vi "register status change event.vi"(11 "generate status number":i32=100) -> (3 "status number":i32)   [LabVIEW 2017, in "testcase-documentation.lvclass"]
uses:
  testcase-documentation.lvclass
  src/user.lib/_NEVSTOP/Communicable State Machine(CSM)/_Support/Priority Queue/Priority Queue.lvclass/Priority Queue.ctl
  f9bca660-bddd-4266-99d8-d96952150cc2.vi
  src/user.lib/_NEVSTOP/Communicable State Machine(CSM)/_Support/Process/CSMP-Sync Call.vi
  src/user.lib/_NEVSTOP/Communicable State Machine(CSM)/Utility/uuid.vi
  src/user.lib/_NEVSTOP/Communicable State Machine(CSM)/Utility/Build Error Cluster.vi
  src/user.lib/_NEVSTOP/Communicable State Machine(CSM)/Utility/Trim Both Whitespace.vi
  src/user.lib/_NEVSTOP/Communicable State Machine(CSM)/AdvanceAPI/CSM - List Modules.vi
  src/user.lib/_NEVSTOP/Communicable State Machine(CSM)/_Support/CSMQ/_CSMObj-Message Check.vi
  src/user.lib/_NEVSTOP/Communicable State Machine(CSM)/_Support/CSMQ/_CSMObj-Enqueue Cross-Module Message.vi
  src/user.lib/_NEVSTOP/Communicable State Machine(CSM)/_Support/CSMQ/_CSMOFGV Get.vi
  src/user.lib/_NEVSTOP/Communicable State Machine(CSM)/_Support/Priority Queue/Enqueue Element.vi
  src/user.lib/_NEVSTOP/Communicable State Machine(CSM)/_Support/Error/CSM No Target Error.vi
  src/user.lib/_NEVSTOP/Communicable State Machine(CSM)/_Support/CSMQ/_CSMOFGV.vi
  src/user.lib/_NEVSTOP/Communicable State Machine(CSM)/_Support/Error/CSM Not Allowed Message.vi
  src/user.lib/_NEVSTOP/Communicable State Machine(CSM)/_Support/Error/CSM Target Error.vi
  src/user.lib/_NEVSTOP/Communicable State Machine(CSM)/_Support/Error/CSM Unhandled State Error.vi
  src/user.lib/_NEVSTOP/Communicable State Machine(CSM)/_Support/Error/CSM Target Timeout Error.vi
  src/user.lib/_NEVSTOP/Communicable State Machine(CSM)/_Support/FGV-BroadcastRegistry/global-CSMQ FGV Change Flag.vi
  src/user.lib/_NEVSTOP/Communicable State Machine(CSM)/Communicable State Machine.lvlib
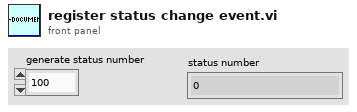
[diagram p1: front panel]
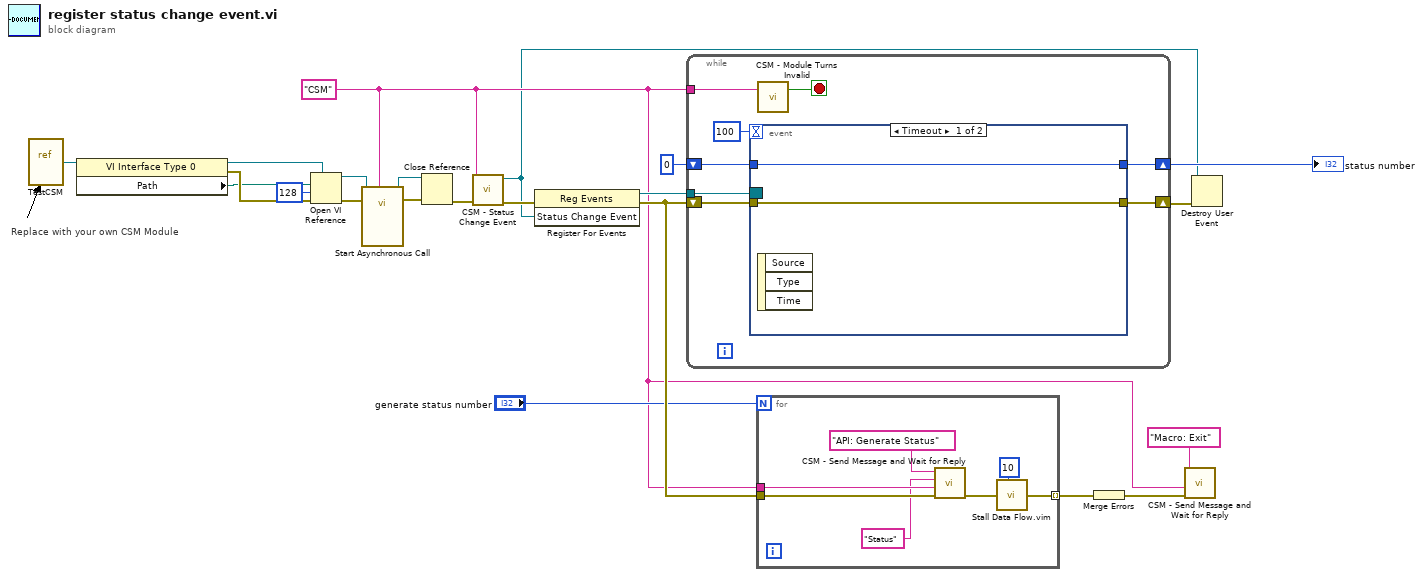
[diagram p0: block diagram]
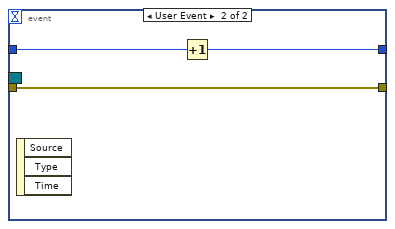
[diagram p2: hidden frame]
diagram:
  w6 = "CSM" ("Name(\"\" to use uuid)")
  # "Replace with your own CSM Module"
  n1 = vi-ref "TestCSM.vi"() -> (w15:refnum<vi>)
  n2 = property class="VI Interface Type 0"(reference=w15) -> (reference out=w19:refnum<vi>, error out=w17:errorcluster, "Path"=w16:path)  [unwired: 1 in]
  n3 = Open VI Reference(type specifier VI Refnum (for type only)=w19, vi path=w16, options=128, error in (no error)=w17) -> (vi reference=w18:refnum<vi>, error out=w14:errorcluster)  [unwired: 2 in]
  n4 = call-by-ref "Start Asynchronous Call"(reference=w18, error in=w14, "Name(\"\" to use uuid)"=w6) -> (reference out=w21:refnum<vi>, error out=w20:errorcluster)  [unwired: 11 in]
  n5 = Close Reference(reference=w21, error in (no error)=w20) -> (error out=w13:errorcluster)
  n6 = call "CSM - Status Change Event.vi"("Error in"=w13, "CSM Module"=w6) -> ("Error out"=w12:errorcluster, "Status Change Event"=w1:refnum<user-event>)  [unwired: 8 in]
  n7 = register-events(error in=w12, w1) -> (reference out=w11:refnum<event-registration>, error out=w10:errorcluster)  [unwired: 1 in]
  n8 = while {
    tunnel: w11 -> [w30]
    tunnel: w6 -> [w27]
    shift-right: [w24] -> w3
    shift-left: 0 -> [w26]
    shift-right: [w23] -> w2
    shift-left: w10 -> [w29]
    stop <- w28 stop-if-true
    n9 = event shown="[0] Timeout" {
      selector: w30 -> [_ _]
      dyn-events: _ -> [_ _]
      timeout: 100 -> [_ _]
      tunnel: w29 -> [w31 w33]
      tunnel: w26 -> [w32 w35]
      tunnel: [w32 w34] -> w24
      tunnel: [w31 w33] -> w23
      event Timeout {
        n10 = event-data() -> ()  [unwired: 1 in, 3 out]
      }
      event User Event {
        n11 = event-data() -> ()  [unwired: 1 in, 3 out]
        n12 = Increment(x=w35) -> (x+1=w34:i32)
      }
    }
    n13 = call "CSM - Module Turns Invalid.vi"("CSM Name"=w27) -> ("Turn Invalid(Exit)?"=w28:bool)  [unwired: 2 in]
  }
  "status number" <- w3
  n14 = for {
    N: "generate status number" -> [_]
    tunnel: w10 -> [w42]
    tunnel: w6 -> [w41]
    tunnel: [w37] -> w8 mode=indexing
    n15 = call "CSM - Send Message and Wait for Reply.vi"("Error In (no error)"=w42, "Target Module"=w41, "Arguments (\"\")"="Status" ("Arguments (\"\")"), "State"="API: Generate Status") -> ("error out"=w38:errorcluster)  [unwired: 5 in, 2 out]
    n16 = call "Stall Data Flow.vim"("value in"=w38, "milliseconds to wait"=10) -> ("value out"=w37:errorcluster)  [unwired: 1 out]
  }
  n17 = Merge Errors(w8) -> (w7:errorcluster)
  n18 = call "CSM - Send Message and Wait for Reply.vi"("Error In (no error)"=w7, "Target Module"=w6, "State"="Macro: Exit") -> ()  [unwired: 6 in, 3 out]
  n19 = Destroy User Event(user event=w1, error in=w2) -> ()  [unwired: 1 out]
